vi "Configure Trigger.vi"(8 "error in (no error)":errorcluster, 9 "trigger holdoff (500.0 E-9 s)":dbl[unit]=5e-07 format="%^.2e", 10 "trigger type (Edge)":i32(ring)=1 items=["Edge"=1, "TV"=5, "Runt"=3, "Glitch"=4, "Width"=2, "AC Line"=7, "Immediate"=6], 11 "CS++Scope":refnum<class "CS++Scope.lvclass">) -> (0 "error out":errorcluster, 3 "CS++Scope out":refnum<class "CS++Scope.lvclass">)   [LabVIEW 2014, in "CS++Scope.lvlib" / "CS++Scope.lvclass"]
doc: "This VI configures the common properties of the trigger subsystem. These properties are the trigger type and holdoff.\nWhen you call IviScope Read Waveform, IviScope Read Waveform Measurement [WM], IviScope Read Min Max Waveform [MmW], or IviScope Initiate Acquisition, the oscilloscope waits for a trigger. You specify the type of trigger for which the oscilloscope waits with the Trigger Type parameter.\nIf the oscilloscope requires multiple waveform acquisitions to build a complete waveform, it waits for the length of time you specify with the Holdoff parameter to elapse since the previous trigger. The oscilloscope then waits for the next trigger. Once the oscilloscope acquires a complete waveform, it returns to the Idle state."
uses:
  CS++Scope.lvclass
  CSPP_Core/Classes/CS++ProcessVariables/ProcessVariable/PV.lvclass
  PV-Enum.ctl
  CSPP_Core/Classes/CS++ProcessVariables/ProcessVariable/PV.lvclass/PV.ctl
  CS++Scope.lvclass/CS++Scope.ctl
  CSPP_Core/Classes/CS++ProcessVariables/ProcessVariable/Write Data.vi
  CSPP_Core/Classes/CS++ProcessVariables/ProcessVariable/Write Timestamp.vi
  CSPP_Core/Classes/CS++ProcessVariables/ProcessVariable/Write Quality.vi
  CSPP_Core/Classes/CS++ProcessVariables/ProcessVariable/Write status.vi
  CSPP_Core/Classes/CS++ProcessVariables/PVConnection/PVConnection.lvclass
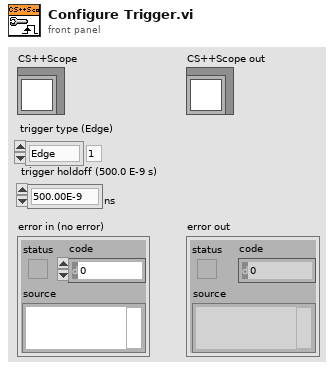
[diagram p1: front panel]
types:
  T1 = typedef "CS++Scope.lvlib/CS++Scope.lvclass/PV-Enum.ctl" = enum16{"ActualSampleRate", "TimePerRecord", "AcquisitionStartTime", "TriggerLevel", "GlitchWidth", "LowReference", "MidReference", "HighReference", "RuntLowThreshold", "RuntHighThreshold", "TriggerHoldoff", "WidthLowThreshold", "WidthHighThreshold", "AcquisitionStatus", "ActualRecordLength", "ActualSampleMode", "ACLineTriggerSlope", "MinRecordLength", "AcquisitionType", "TriggerSlope", "GlitchCondition", "GlitchPolarity", "InterpolationMethod", "NumberOfAverages", "NumberOfEnvelopes", "TriggerType", "TriggerCoupling", "TriggerModifier", "TVLineNumber", "TVEvent", "TVTriggerPolarity", "TVSignalFormat", "WidthCondition", "WidthPolarity", "MeasurementDone", "ContinousAcquisition", "TriggerSource", "Waveform", "ActualTimeIncrement"}
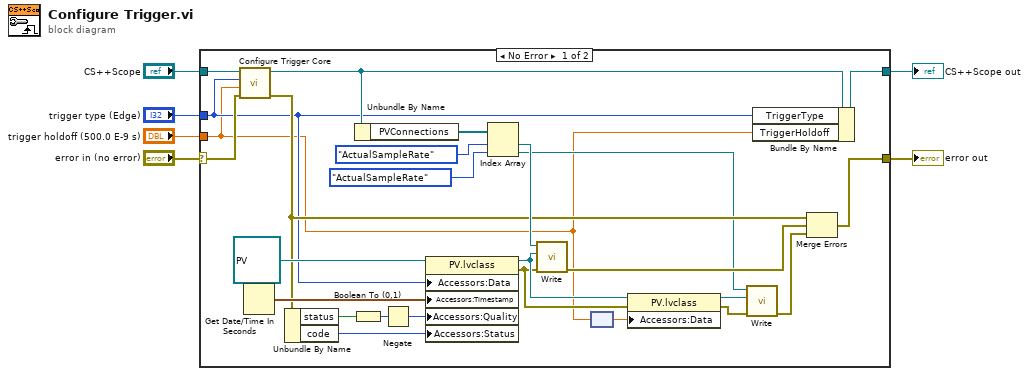
[diagram p0: block diagram]
diagram:
  n1 = case shown="No Error" "error in (no error)" {
    selector: "error in (no error)" -> [w10 w34]
    tunnel: [w11 w34] -> w5
    tunnel: [w12 w33] -> w2
    tunnel: "CS++Scope" -> [w13 w33]
    tunnel: "trigger type (Edge)" -> [w9 _]
    tunnel: "trigger holdoff (500.0 E-9 s)" -> [w8 _]
    frame No Error {
      n2 = call-dynamic "Configure Trigger Core.vi"("error in (no error)"=w10, "trigger holdoff (500.0 E-9 s)"=w8, "trigger type (Edge)"=w9, "CS++Scope"=w13) -> ("error out"=w21:errorcluster, "CS++Scope out"=w22:refnum<class "CS++Scope.lvclass">)  [unwired: 6 in]
      n3 = Get Date/Time In Seconds() -> (seconds since 1Jan1904=w27:timestamp)
      n4 = Unbundle By Name(w21) -> ("status"=w30:bool, "code"=w31:i32)
      n5 = Boolean To (0,1)(Boolean=w30) -> (0, 1=w29:i16)
      n6 = Unbundle By Name(w22) -> ("PVConnections"=w26:refnum<class "PVConnection.lvclass">[])
      n7 = Negate(x=w29) -> (-x=w28:i16)
      n8 = property class="PV.lvclass"(reference=refnum<class "PV.lvclass"> refnum ("CS++ProcessVariables.lvlib:PV.lvclass"), "Accessors:Data"=w9, "Accessors:Timestamp"=w27, "Accessors:Quality"=w28, "Accessors:Status"=w31) -> (reference out=w18:refnum<class "PV.lvclass">, error out=w14:errorcluster)  [unwired: 1 in]
      n9 = Index Array(array=w26, index #1=PV-Enum."ActualSampleRate" ("PV-Enum"), index #2=PV-Enum."ActualSampleRate" ("PV-Enum")) -> (element #1=w24:refnum<class "PVConnection.lvclass">, element #2=w16:refnum<class "PVConnection.lvclass">)
      n10 = call "Write.vi"("error in (no error)"=w14, "PV"=w18, "PVConnection in"=w24) -> ("error out"=w23:errorcluster)  [unwired: 7 in, 1 out]
      n11 = node(w8) -> (w7:dbl)
      n12 = property class="PV.lvclass"(reference=w18, error in=w14, "Accessors:Data"=w7) -> (reference out=w15:refnum<class "PV.lvclass">, error out=w17:errorcluster)
      n13 = call "Write.vi"("error in (no error)"=w17, "PV"=w15, "PVConnection in"=w16) -> ("error out"=w19:errorcluster)  [unwired: 7 in, 1 out]
      n14 = Bundle By Name(cluster=w22, "TriggerType"=w9, "TriggerHoldoff"=w8) -> (w12:refnum<class "CS++Scope.lvclass">)
      n15 = Merge Errors(w21, w23, w19) -> (w11:errorcluster)
    }
    frame Error {
    }
  }
  "error out" <- w5
  "CS++Scope out" <- w2
